vi "Create Vertical Toolbar.vi"(8 "error in (no error)":errorcluster, 10 "Button Over Index":i32, 11 "Toolbar Control in":refnum<class "Toolbar Control.lvclass">) -> (0 "error out":errorcluster)   [LabVIEW 2011, in "Toolbar Control.lvclass"]
doc: "This VI will create the Vertical Toolbar menu and run it.\n\n-------------\nDeveloped by Brian Hoover (hooovahh)"
uses:
  Toolbar Control.lvclass
  Toolbar Control.lvclass/Toolbar Control.ctl
  Vertical Toolbar Dialog.vi
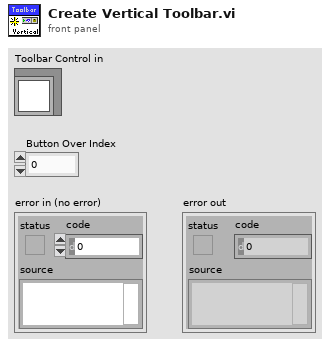
[diagram p1: front panel]
types:
  T1 = typedef "Toolbar Control.lvclass/Icon Data.ctl" = cluster{"Original Image Path":path, "Original Image Data":T2, "Scaled Icon":picture, "Button Name":string, "Button State":T3, "Icon Type":T4}
  T2 = typedef "imagedata.ctl" = cluster{"image type":i32, "image depth":i32, "image":u8[], "mask":u8[], "colors":u32[], "Rectangle":cluster{"left":i16, "top":i16, "right":i16, "bottom":i16}}
  T3 = typedef "Toolbar Control.lvclass/Button State.ctl" = enum8{"Enabled", "Disabled", "Disabled and Grayed Out"}
  T4 = typedef "Icon Type.ctl" = enum16{"Normal Icon", "Separator Icon", "More Options"}
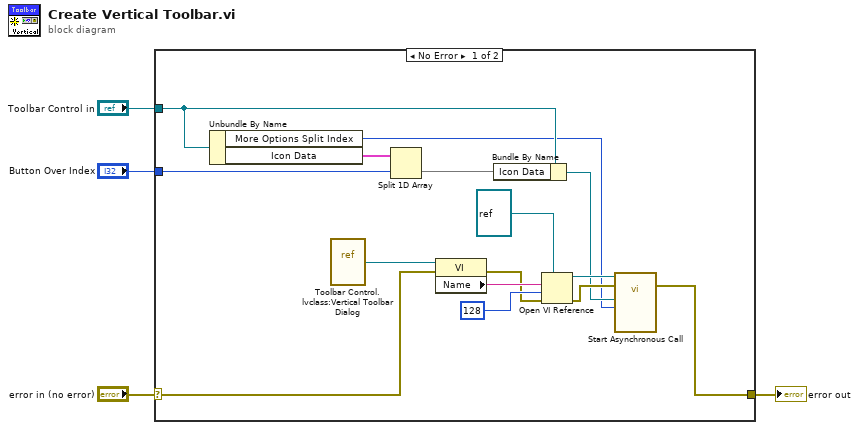
[diagram p0: block diagram]
diagram:
  n1 = case shown="No Error" "error in (no error)" {
    selector: "error in (no error)" -> [w12 w20]
    tunnel: [w14 w20] -> w3
    tunnel: "Toolbar Control in" -> [w7 _]
    tunnel: "Button Over Index" -> [w9 _]
    frame No Error {
      n2 = Unbundle By Name(w7) -> ("More Options Split Index"=w5:i32, "Icon Data"=w10:T1[])
      n3 = vi-ref "Toolbar Control.lvclass:Vertical Toolbar Dialog.vi"() -> (w19:refnum<vi>)
      n4 = Split 1D Array(array=w10, index=w9) -> (second subarray=w8:T1[])  [unwired: 1 out]
      n5 = property class="VI"(reference=w19, error in=w12) -> (error out=w13:errorcluster, "Name"=w18:string)  [unwired: 1 out]
      n6 = Bundle By Name(cluster=w7, "Icon Data"=w8) -> (w6:refnum<class "Toolbar Control.lvclass">)
      n7 = Open VI Reference(type specifier VI Refnum (for type only)=refnum<vi> refnum, vi path=w18, options=128, error in (no error)=w13) -> (vi reference=w16:refnum<vi>, error out=w11:errorcluster)  [unwired: 2 in]
      n8 = call-by-ref "Start Asynchronous Call"(reference=w16, error in=w11, "More Options Split Index"=w5, "Toolbar Control in"=w6) -> (error out=w14:errorcluster)  [unwired: 10 in, 1 out]
    }
    frame Error {
    }
  }
  "error out" <- w3
